vi "Mutex Attr Delete Object.vi"(8 "error in (no error)":errorcluster, 11 "Mutex Attr in":T1) -> (0 "error out":errorcluster, 3 "mutex attr pointer out":u64)   [LabVIEW 2013, in "POSIX Threads.lvlib" / "Mutex Attr.lvclass"]
doc: "Destroys the LabVIEW object used to encapsulate a pthread mutex attribute object."
uses:
  Mutex Attr.lvclass
  Controls/reference.ctl
  POSIX Thread Object/POSIX Thread Object.lvclass/POSIX Thread Object.ctl
  POSIX Thread Object/POSIX Thread Object.lvclass
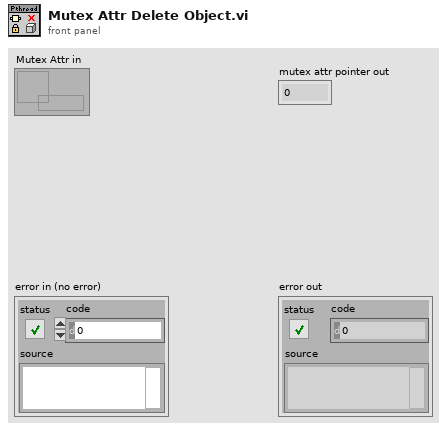
[diagram p1: front panel]
types:
  T1 = typedef "POSIX Threads.lvlib/Mutex Attr.lvclass/reference.ctl" = refnum<data-value>
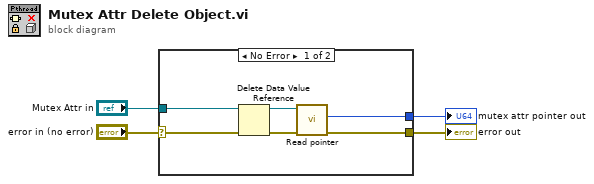
[diagram p0: block diagram]
diagram:
  n1 = case shown="No Error" "error in (no error)" {
    selector: "error in (no error)" -> [w8 w11]
    tunnel: [w6 w11] -> w3
    tunnel: "Mutex Attr in" -> [w7 _]
    tunnel: [w5 _] -> w1
    frame No Error {
      n2 = Delete Data Value Reference(data value reference=w7, error in=w8) -> (data value=w10:refnum<class "Mutex Attr.lvclass">, error out=w9:errorcluster)
      n3 = call "Read pointer.vi"("error in (no error)"=w9, "POSIX Thread Object in"=w10) -> ("error out"=w6:errorcluster, "pointer"=w5:u64)  [unwired: 7 in, 1 out]
    }
    frame Error {
    }
  }
  "error out" <- w3
  "mutex attr pointer out" <- w1
